vi "1L21_Rm_Iref.vi"(8 "I ref":dbl=0.001, 11 "Vm":dbl) -> (3 "Rm":dbl)   [LabVIEW 2010, in "lv_01.lvlib"]
uses:
  lv_01.lvlib
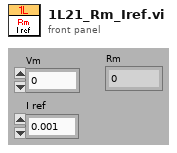
[diagram p1: front panel]
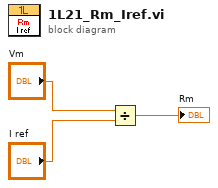
[diagram p0: block diagram]
diagram:
  n1 = Divide(x="Vm", y="I ref") -> (x/y=→"Rm":dbl)
